vi "DAC Configure.vi"(8 "error in":errorcluster, 11 "DAC Inclino in":refnum<class "DAC Inclinometer.lvclass">) -> (0 "error out":errorcluster, 3 "DAC Inclino out":refnum<class "DAC Inclinometer.lvclass">)   [LabVIEW 2019, in "DAC.lvlib" / "DAC Inclinometer.lvclass"]
uses:
  DAC Inclinometer.lvclass
  C:/Users/krio/Documents/LV_Projects/test-stand/App/DAC/DAC.lvclass
  DAC.lvclass/DAC.ctl
  DAC Inclinometer.lvclass/DAC Inclinometer.ctl
  <vilib>/DAQmx/create/channels.llb/DAQmx Create Channel (AI-Voltage-Basic).vi
  DAC.lvclass
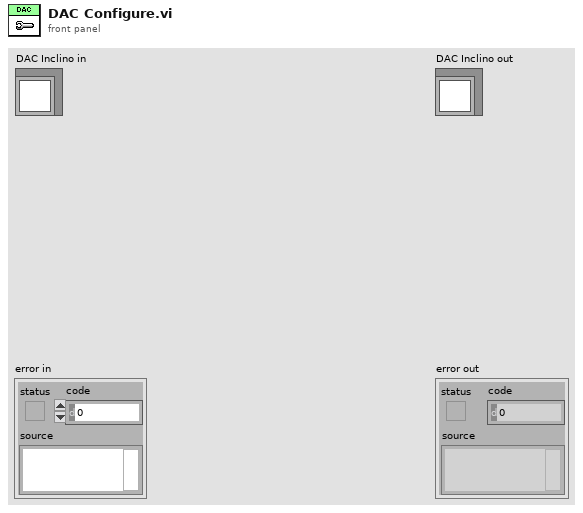
[diagram p1: front panel]
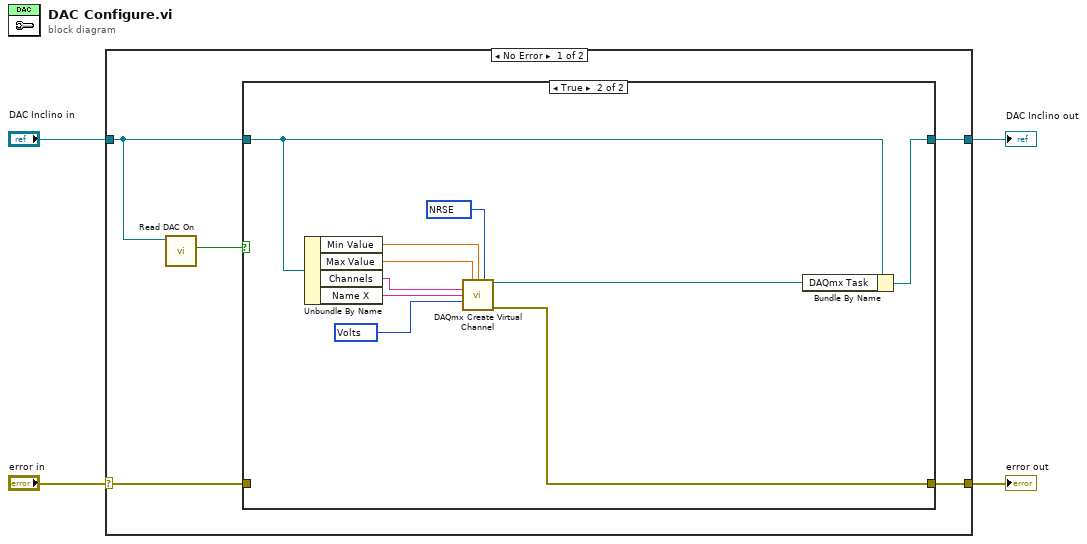
[diagram p0: block diagram]
diagram:
  n1 = case shown="No Error" "error in" {
    selector: "error in" -> [w6 w23]
    tunnel: [w5 w23] -> w4
    tunnel: [w7 w22] -> w3
    tunnel: "DAC Inclino in" -> [w9 w22]
    frame No Error {
      n2 = call "Read DAC On.vi"("DAC in"=w9) -> ("DAC On"=w8:bool)  [unwired: 8 in, 2 out]
      n3 = case shown="True" w8 {
        tunnel: w9 -> [w11 w20]
        tunnel: [w11 w19] -> w7
        tunnel: w6 -> [w10 _]
        tunnel: [w10 w15] -> w5
        frame False {
          # "Temperature measurement is off."
        }
        frame True {
          w13 = 10078 items=["Default"=-1, "RSE"=10083, "NRSE"=10078, "Differential"=10106, "Pseudodifferential"=12529] ("input terminal configuration")
          w14 = 10348 items=["Volts"=10348, "From Custom Scale"=10065] ("units")
          # "Temperature measurement is on."
          n4 = Unbundle By Name(w20) -> ("Min Value"=w17:dbl, "Max Value"=w21:dbl, "Channels"=w12:string, "Name X"=w18:string)
          n5 = call-poly <vilib>:"DAQmx Create Virtual Channel.vi"("maximum value"=w21, "minimum value"=w17, "input terminal configuration"=w13, "physical channels"=w12, "name to assign"=w18, "units"=w14) -> ("task out"=w16:refnum<k21>, "error out"=w15:errorcluster)  [unwired: 8 in]
          n6 = Bundle By Name(cluster=w20, "DAQmx Task"=w16) -> (w19:refnum<class "DAC Inclinometer.lvclass">)
        }
      }
    }
    frame Error {
    }
  }
  "error out" <- w4
  "DAC Inclino out" <- w3
